vi "TriggerBoxActor.vi"() -> ()   [LabVIEW 2013, in "TriggerBox.lvclass"]
uses:
  TriggerBox.lvclass
  FPGATargetClass/FPGATarget.lvclass
panel:
  out "TriggerBox out":refnum<class "TriggerBox.lvclass">
  out "error out":errorcluster
  in  "error in":errorcluster
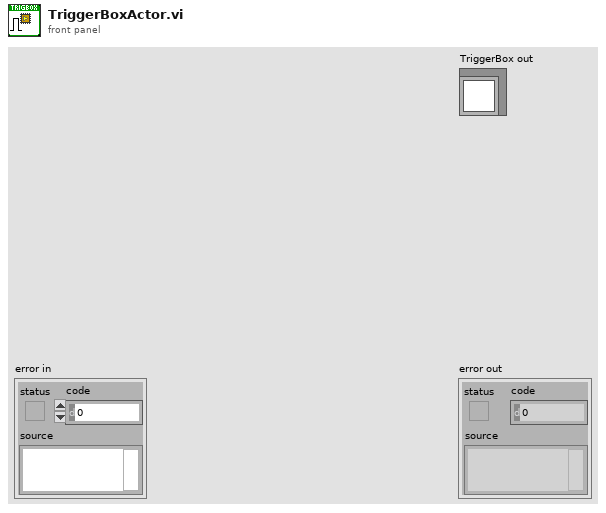
[diagram p1: front panel]
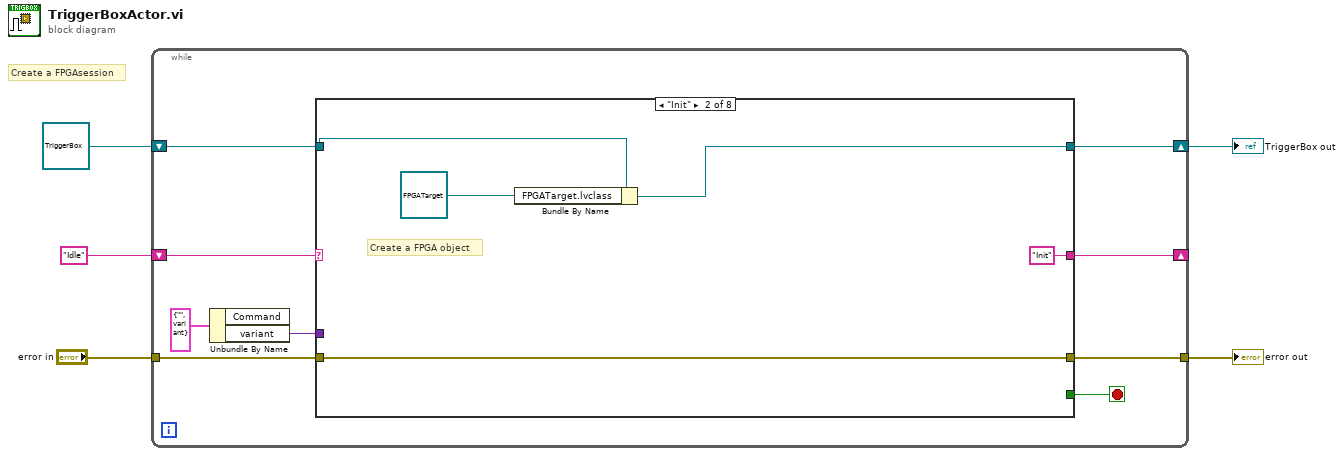
[diagram p0: block diagram]
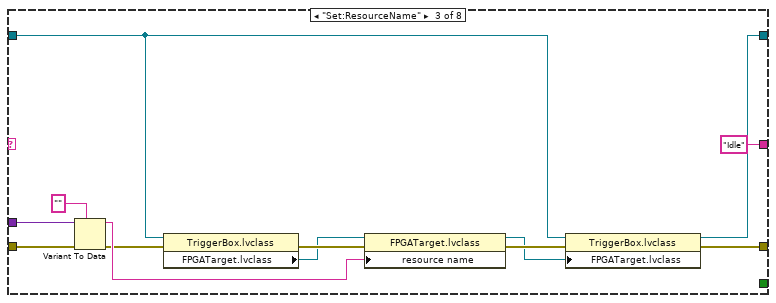
[diagram p3: hidden frame]
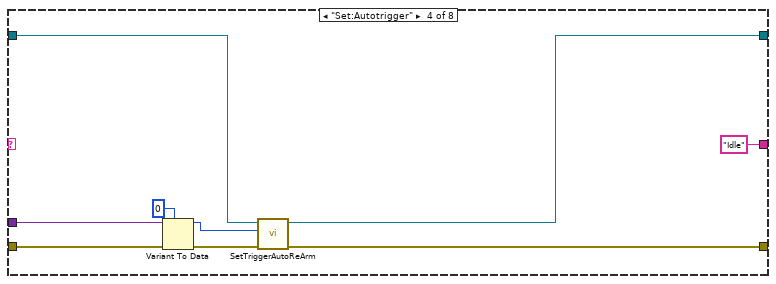
[diagram p4: hidden frame]
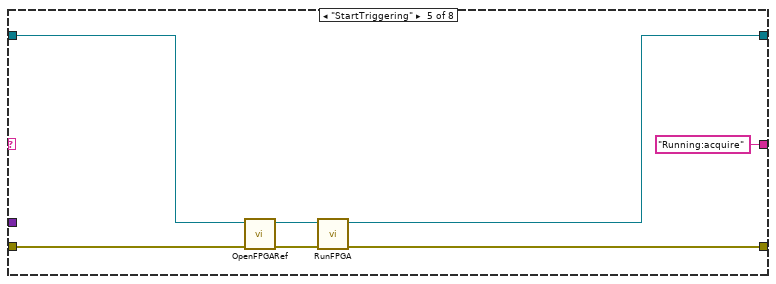
[diagram p5: hidden frame]
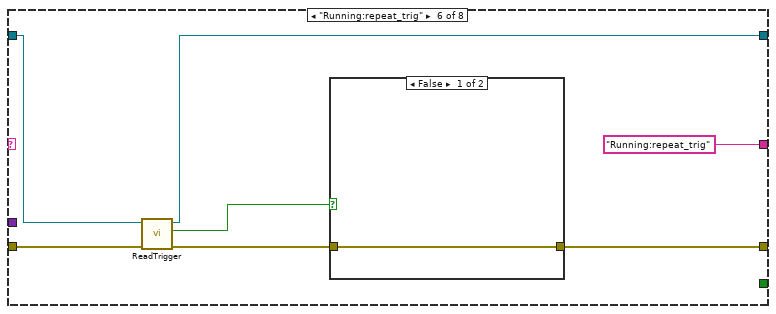
[diagram p6: hidden frame]
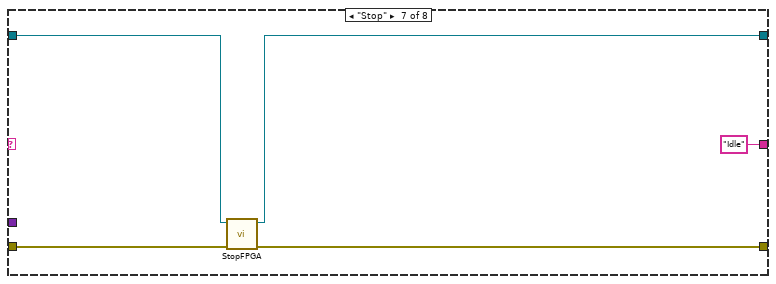
[diagram p8: hidden frame]
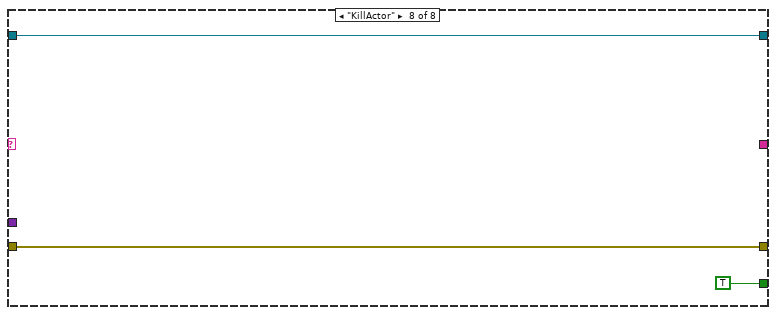
[diagram p9: hidden frame]
diagram:
  # "Create a FPGAsession"
  n1 = while {
    tunnel: "error in" -> [w14]
    tunnel: [w13] -> w4
    shift-right: [w10] -> _
    shift-left: "Idle" -> [w12]
    shift-right: [w9] -> w1
    shift-left: refnum<class "TriggerBox.lvclass"> refnum ("HWTriggerDetector.lvclass") -> [w11]
    stop <- w8 stop-if-true
    n2 = Unbundle By Name(cluster{"Command":string, "variant":variant} {"Command"="", "variant"=variant}) -> ("variant"=w6:variant)  [unwired: 1 out]
    n3 = case shown="\"Init\"" w12 {
      selector: w12 -> [w15 _ _ _ _ _ _ _]
      tunnel: w14 -> [w17 w20 w32 w44 w46 w58 w65 w66]
      tunnel: [w17 w20 w31 w38 w51 w55 w64 w66] -> w13
      tunnel: w11 -> [w16 w22 w26 w40 w45 w52 w63 w68]
      tunnel: [w16 w19 w27 w41 w48 w53 w62 w68] -> w9
      tunnel: [w15 "Init" "Idle" "Idle" "Running:acquire" "Running:repeat_trig" "Idle" _] -> w10
      tunnel: [_ _ _ _ _ _ _ TRUE] -> w8
      tunnel: w6 -> [_ _ w30 w43 _ _ _ _]
      frame Default {
      }
      frame "Init" {
        # "Create a FPGA object"
        n4 = Bundle By Name(cluster=w22, "FPGATarget.lvclass"=refnum<class "FPGATarget.lvclass"> refnum) -> (w19:refnum<class "TriggerBox.lvclass">)
      }
      frame "Set:ResourceName" {
        n5 = Variant To Data(error in=w32, type="", Variant=w30) -> (data=w33:string, error out=w25:errorcluster)
        n6 = property class="TriggerBox.lvclass"(reference=w26, error in=w25) -> (error out=w24:errorcluster, "FPGATarget.lvclass"=w23:refnum<class "FPGATarget.lvclass">)  [unwired: 1 out]
        n7 = property class="FPGATarget.lvclass"(reference=w23, error in=w24, "resource name"=w33) -> (reference out=w28:refnum<class "FPGATarget.lvclass">, error out=w35:errorcluster)
        n8 = property class="TriggerBox.lvclass"(reference=w26, error in=w35, "FPGATarget.lvclass"=w28) -> (reference out=w27:refnum<class "TriggerBox.lvclass">, error out=w31:errorcluster)
      }
      frame "Set:Autotrigger" {
        n9 = Variant To Data(error in=w44, type=i64 0 ("TriggerAutoReArm"), Variant=w43) -> (data=w36:i64, error out=w39:errorcluster)
        n10 = call-dynamic "SetTriggerAutoReArm.vi"("error in"=w39, "TriggerAutoReArm(mSec)"=w36, "TriggerBox in"=w40) -> ("error out"=w38:errorcluster, "TriggerBox out"=w41:refnum<class "TriggerBox.lvclass">)  [unwired: 7 in]
      }
      frame "StartTriggering" {
        n11 = call-dynamic "OpenFPGARef.vi"("error in"=w46, "FPGASession in"=w45) -> ("error out"=w49:errorcluster, "FPGASession out"=w50:refnum<class "TriggerBox.lvclass">)  [unwired: 8 in]
        n12 = call-dynamic "RunFPGA.vi"("error in"=w49, "FPGASession in"=w50) -> ("error out"=w51:errorcluster, "FPGASession out"=w48:refnum<class "TriggerBox.lvclass">)  [unwired: 8 in]
      }
      frame "Running:repeat_trig" {
        n13 = call-dynamic "ReadTrigger.vi"("error in"=w58, "TriggerBox in"=w52) -> ("error out"=w56:errorcluster, "TriggerFired"=w57:bool, "TriggerBox out"=w53:refnum<class "TriggerBox.lvclass">)  [unwired: 6 in, 1 out]
        n14 = case shown="False" w57 {
          tunnel: w56 -> [w59 w60]
          tunnel: [w59 w60] -> w55
          frame False {
          }
          frame True {
          }
        }
      }
      frame "Stop" {
        n15 = call-dynamic "StopFPGA.vi"("error in"=w65, "FPGASession in"=w63) -> ("error out"=w64:errorcluster, "FPGASession out"=w62:refnum<class "TriggerBox.lvclass">)  [unwired: 8 in]
      }
      frame "KillActor" {
      }
    }
  }
  "error out" <- w4
  "TriggerBox out" <- w1
